vi "LWESP301_Example.vi"() -> ()   [LabVIEW 2010]
uses:
  C:/PVCS/IHM_Visual_Studio_NET/MotionControl/ESP301/Distribution/LabView/Source code/Dll/Newport.ESP301.CommandInterface.DLL
  Dll/Newport.ESP301.CommandInterface.DLL
panel:
  out "errstring (HN)":string
  out "HN_Set error":i32
  out "LC0_Set error":i32
  out "VE error":i32
  out "LC2_Set error":i32
  out "errstring (LC0)":string
  out "errstring (VE)":string
  out "Error out":errorcluster caption="error out"
  in  "Instrument Key":string
  out "errstring (LC2)":string
  out "ControllerVersion":string
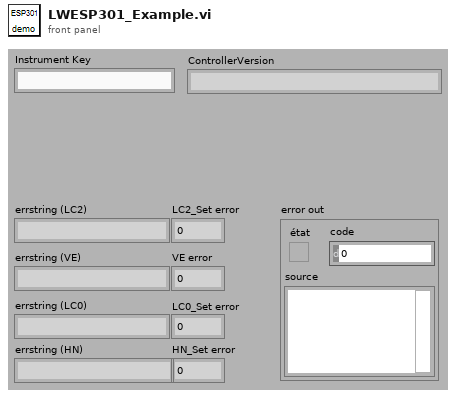
[diagram p1: front panel]
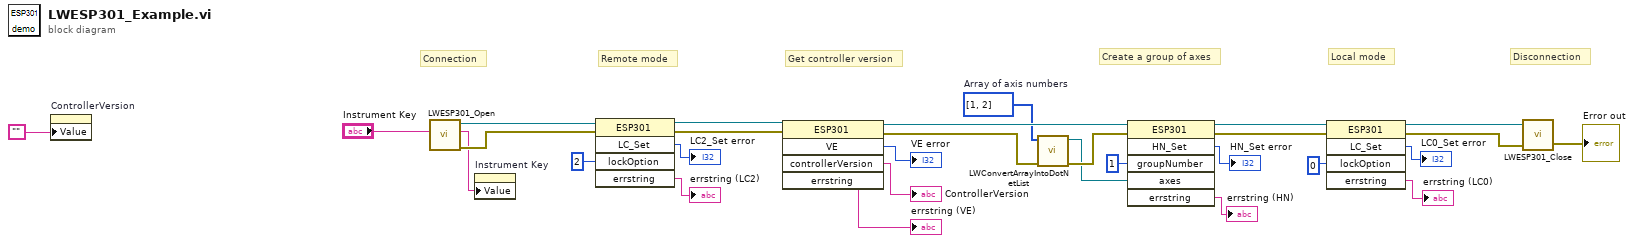
[diagram p0: block diagram]
diagram:
  w14 = i32[] [1, 2]  # Array of axis numbers
  # "Create a group of axes"
  # "Get controller version"
  # "Local mode"
  # "Remote mode"
  # "Disconnection"
  # "Connection"
  n1 = property on="ControllerVersion" class="Ch"("Value"="") -> ()  [unwired: 2 in, 2 out]
  n2 = call "LWESP301_Open.vi"("Instrument Key IN"="Instrument Key") -> ("error out"=w25:errorcluster, "Instrument Key OUT"=w12:string, "ESP301 Reference"=w28:refnum<k24>)  [unwired: 3 in, 1 out]
  n3 = property on="Instrument Key" class="Ch"("Value"=w12) -> ()  [unwired: 2 in, 2 out]
  n4 = invoke class="ESP301" method="LC_Set"(reference=w28, error in=w25, "lockOption"=2 ("program")) -> (reference out=w27:refnum<k24>, error out=w26:errorcluster, "LC_Set"=→"LC2_Set error":i32, "errstring"=→"errstring (LC2)":string)  [unwired: 2 in, 1 out]
  n5 = invoke on="Nœud de méthode" class="ESP301" method="VE"(reference=w27, error in=w26) -> (reference out=w16:refnum<k24>, error out=w15:errorcluster, "VE"=→"VE error":i32, "controllerVersion"=→"ControllerVersion":string, "errstring"=→"errstring (VE)":string)  [unwired: 3 in]
  n6 = call "LWConvertArrayIntoDotNetList.vi"("Error IN"=w15, "array of axes"=w14) -> ("Error OUT"=w13:errorcluster, "\"axes\" List"=w5:refnum<k24>)  [unwired: 8 in]
  n7 = invoke class="ESP301" method="HN_Set"(reference=w16, error in=w13, "groupNumber"=1, "axes"=w5) -> (reference out=w19:refnum<k24>, error out=w18:errorcluster, "HN_Set"=→"HN_Set error":i32, "errstring"=→"errstring (HN)":string)  [unwired: 2 in, 2 out]
  n8 = invoke class="ESP301" method="LC_Set"(reference=w19, error in=w18, "lockOption"=0) -> (reference out=w24:refnum<k24>, error out=w23:errorcluster, "LC_Set"=→"LC0_Set error":i32, "errstring"=→"errstring (LC0)":string)  [unwired: 2 in, 1 out]
  n9 = call "LWESP301_Close.vi"("error in (no error)"=w23, "ESP301 Reference"=w24) -> ("Error out"=→"Error out":errorcluster)  [unwired: 2 in]
